vi "SwerveDriveCalculations.vi"(11 "SwerveCommands":dbl[](array[numeric])) -> ()   [LabVIEW 2016]
panel:
  out "Velocity":dbl[](array[numeric])
  out "Angle":dbl[](array[numeric])
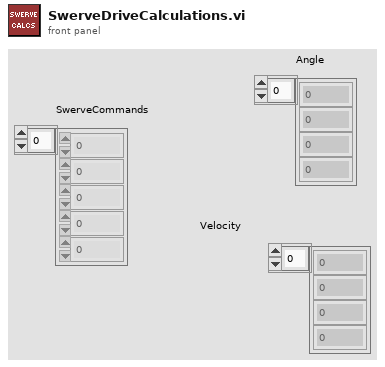
[diagram p1: front panel]
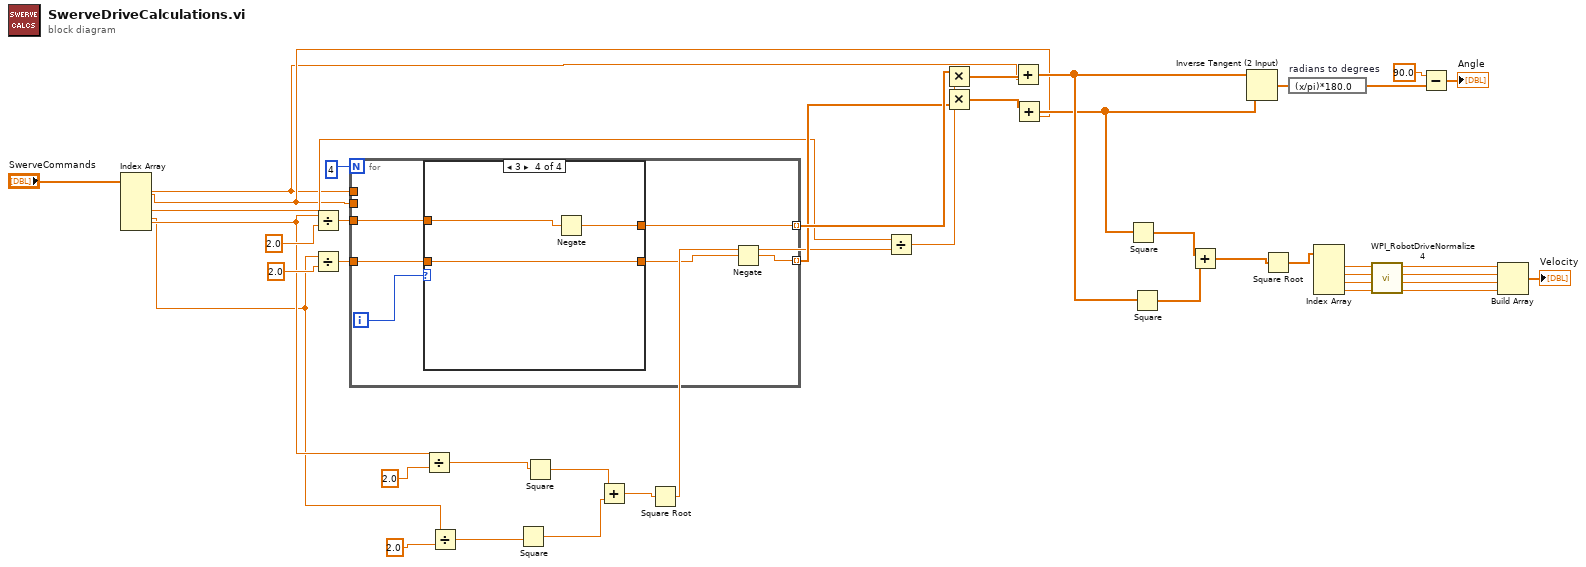
[diagram p0: block diagram]
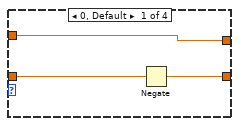
[diagram p2: hidden frame]
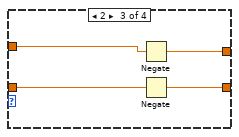
[diagram p4: hidden frame]
diagram:
  n1 = Index Array(array="SwerveCommands") -> (element #1=w4:dbl, element #2=w3:dbl, element #3=w17:dbl, element #4=w1:dbl, element #5=w2:dbl)  [unwired: 5 in]
  n2 = Divide(x=w2, y=2.0) -> (x/y=w33:dbl)
  n3 = Divide(x=w1, y=2.0) -> (x/y=w32:dbl)
  n4 = for {
    N: 4 -> [_]
    tunnel: w33 -> [w47]
    tunnel: w32 -> [w46]
    tunnel: w3 -> [_]
    tunnel: w4 -> [_]
    tunnel: [w44] -> w22 mode=indexing
    tunnel: [w43] -> w23 mode=indexing
    i -> [w48]
    n5 = case shown="3" w48 {
      tunnel: w47 -> [w49 w52 w57 w60]
      tunnel: w46 -> [w51 w53 w55 w58]
      tunnel: [w50 w53 w54 w58] -> w45
      tunnel: [w49 w52 w56 w59] -> w43
      frame 0, Default {
        n6 = Negate(x=w51) -> (-x=w50:dbl)
      }
      frame 1 {
      }
      frame 2 {
        n7 = Negate(x=w57) -> (-x=w56:dbl)
        n8 = Negate(x=w55) -> (-x=w54:dbl)
      }
      frame 3 {
        n9 = Negate(x=w60) -> (-x=w59:dbl)
      }
    }
    n10 = Negate(x=w45) -> (-x=w44:dbl)
  }
  n11 = Divide(x=w2, y=2.0) -> (x/y=w28:dbl)
  n12 = Divide(x=w1, y=2.0) -> (x/y=w29:dbl)
  n13 = Square(x=w29) -> (x^2=w26:dbl)
  n14 = Square(x=w28) -> (x^2=w27:dbl)
  n15 = Add(x=w27, y=w26) -> (x+y=w25:dbl)
  n16 = Square Root(x=w25) -> (sqrt(x)=w5:dbl)
  n17 = Divide(x=w17, y=w5) -> (x/y=w24:dbl)
  n18 = Multiply(x=w23, y=w24) -> (x*y=w16:dbl[])
  n19 = Multiply(x=w24, y=w22) -> (x*y=w15:dbl[])
  n20 = Add(x=w16, y=w3) -> (x+y=w14:dbl[])
  n21 = Add(x=w15, y=w4) -> (x+y=w13:dbl[])
  n22 = Square(x=w13) -> (x^2=w12:dbl[])
  n23 = Square(x=w14) -> (x^2=w11:dbl[])
  n24 = Add(x=w12, y=w11) -> (x+y=w10:dbl[])
  n25 = Inverse Tangent (2 Input)(1:w13, 2:w14) -> (0:w20:dbl[])
  n26 = Square Root(x=w10) -> (sqrt(x)=w9:dbl[])
  n27 = expression code="(x/pi)*180.0" "radians to degrees"(w20) -> (w19:dbl[])
  n28 = Index Array(array=w9) -> (element #1=w8:dbl, element #3=w6:dbl, element #4=w7:dbl)  [unwired: 4 in, 1 out]
  n29 = call <vilib>:"WPI_RobotDriveNormalize 4.vi"("D"=w7, "C"=w6, "B"=w8, "A"=w8) -> ("D'"=w40:dbl, "C'"=w39:dbl, "B'"=w38:dbl, "A'"=w37:dbl)
  n30 = Subtract(x=90.0, y=w19) -> (x-y=→"Angle":dbl[])
  n31 = Build Array(w37, w38, w39, w40) -> (→"Velocity":dbl[])
